vi "ProductionBoardReduction.vi"(11 "ProductionBoard":T3={"StartHour"=[{"Hour"=5, "Minute"=0}, {"Hour"=6, "Minute"=0}, {"Hour"=7, "Minute"=0}, {"Hour"=7, "Minute"=30}, {"Hour"=0, "Minute"=0}, {"Hour"=0, "Minute"=0}, {"Hour"=0, "Minute"=0}, {"Hour"=0, "Minute"=0}, {"Hour"=0, "Minute"=0}], "Goal"=[], "EndHour"=[{"Hour"=5, "Minute"=59}, {"Hour"=6, "Minute"=59}, {"Hour"=7, "Minute"=10}, {"Hour"=7, "Minute"=59}, {"Hour"=0, "Minute"=0}, {"Hour"=0, "Minute"=0}, {"Hour"=0, "Minute"=0}, {"Hour"=0, "Minute"=0}, {"Hour"=0, "Minute"=0}], "AM/PM"=[{"AM/PM"=0}, {"AM/PM"=0}, {"AM/PM"=0}, {"AM/PM"=0}, {"AM/PM"=0}, {"AM/PM"=0}, {"AM/PM"=0}, {"AM/PM"=0}, {"AM/PM"=0}], "Actual"=[], "%"=[], "Status"=[], "Comments"=[]} {"AM/PM"."AM/PM" items=["AM", "PM"]; "EndHour"."Minute" items=["00", "1", "2", "3", "4", "5", "6", "7", "8", "9", "10", "11", "12", "13", "14", "15", "16", "17", "18", "19", "20", "21", "22", "23", "24", "25", "26", "27", "28", "29", "30", "31", "32", "33", "34", "35", "36", "37", "38", "39", "40", "41", "42", "43", "44", "45", "46", "47", "48", "49", "50", "51", "52", "53", "54", "55", "56", "57", "58", "59"]; "EndHour"."Hour" items=["00", "1", "2", "3", "4", "5", "6", "7", "8", "9", "10", "11", "12", "13", "14", "15", "16", "17", "18", "19", "20", "21", "22", "23"]; "StartHour"."Minute" items=["00", "1", "2", "3", "4", "5", "6", "7", "8", "9", "10", "11", "12", "13", "14", "15", "16", "17", "18", "19", "20", "21", "22", "23", "24", "25", "26", "27", "28", "29", "30", "31", "32", "33", "34", "35", "36", "37", "38", "39", "40", "41", "42", "43", "44", "45", "46", "47", "48", "49", "50", "51", "52", "53", "54", "55", "56", "57", "58", "59"]; "StartHour"."Hour" items=["00", "1", "2", "3", "4", "5", "6", "7", "8", "9", "10", "11", "12", "13", "14", "15", "16", "17", "18", "19", "20", "21", "22", "23"]}) -> (3 "CloudProductionBoard":T2(array[cluster]) {"EndMinute" items=["00", "1", "2", "3", "4", "5", "6", "7", "8", "9", "10", "11", "12", "13", "14", "15", "16", "17", "18", "19", "20", "21", "22", "23", "24", "25", "26", "27", "28", "29", "30", "31", "32", "33", "34", "35", "36", "37", "38", "39", "40", "41", "42", "43", "44", "45", "46", "47", "48", "49", "50", "51", "52", "53", "54", "55", "56", "57", "58", "59"]; "EndHour" items=["00", "1", "2", "3", "4", "5", "6", "7", "8", "9", "10", "11", "12", "13", "14", "15", "16", "17", "18", "19", "20", "21", "22", "23"]; "InitialMinute" items=["00", "1", "2", "3", "4", "5", "6", "7", "8", "9", "10", "11", "12", "13", "14", "15", "16", "17", "18", "19", "20", "21", "22", "23", "24", "25", "26", "27", "28", "29", "30", "31", "32", "33", "34", "35", "36", "37", "38", "39", "40", "41", "42", "43", "44", "45", "46", "47", "48", "49", "50", "51", "52", "53", "54", "55", "56", "57", "58", "59"]; "InitialHour" items=["00", "1", "2", "3", "4", "5", "6", "7", "8", "9", "10", "11", "12", "13", "14", "15", "16", "17", "18", "19", "20", "21", "22", "23"]})   [LabVIEW 2017]
panel:
  out "ProductionHour":T1 {"EndMinute" items=["00", "1", "2", "3", "4", "5", "6", "7", "8", "9", "10", "11", "12", "13", "14", "15", "16", "17", "18", "19", "20", "21", "22", "23", "24", "25", "26", "27", "28", "29", "30", "31", "32", "33", "34", "35", "36", "37", "38", "39", "40", "41", "42", "43", "44", "45", "46", "47", "48", "49", "50", "51", "52", "53", "54", "55", "56", "57", "58", "59"]; "EndHour" items=["00", "1", "2", "3", "4", "5", "6", "7", "8", "9", "10", "11", "12", "13", "14", "15", "16", "17", "18", "19", "20", "21", "22", "23"]; "InitialMinute" items=["00", "1", "2", "3", "4", "5", "6", "7", "8", "9", "10", "11", "12", "13", "14", "15", "16", "17", "18", "19", "20", "21", "22", "23", "24", "25", "26", "27", "28", "29", "30", "31", "32", "33", "34", "35", "36", "37", "38", "39", "40", "41", "42", "43", "44", "45", "46", "47", "48", "49", "50", "51", "52", "53", "54", "55", "56", "57", "58", "59"]; "InitialHour" items=["00", "1", "2", "3", "4", "5", "6", "7", "8", "9", "10", "11", "12", "13", "14", "15", "16", "17", "18", "19", "20", "21", "22", "23"]}
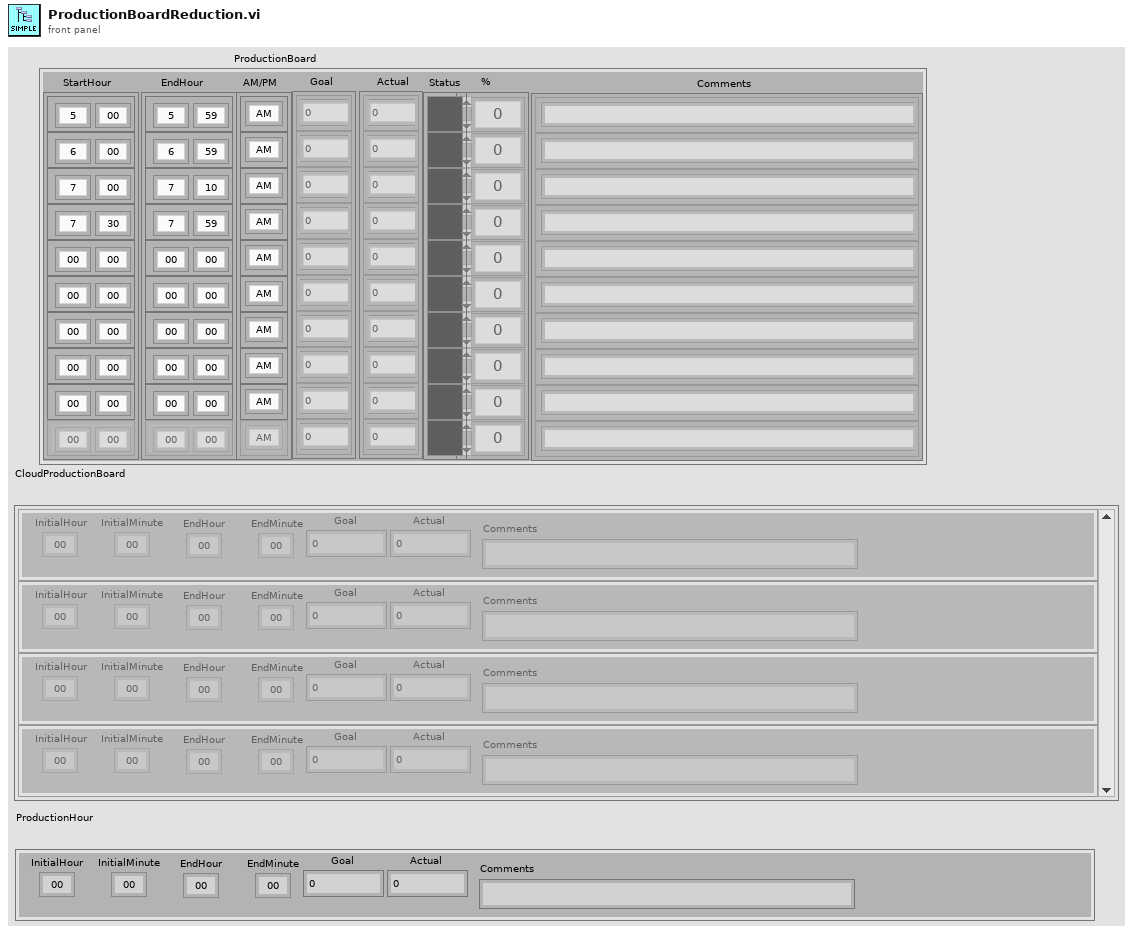
[diagram p1: front panel]
types:
  T1 = cluster{"InitialHour":u16, "InitialMinute":u16, "EndHour":u16, "EndMinute":u16, "Goal":dbl, "Actual":dbl, "Comments":string}
  T2 = cluster{"InitialHour":u16, "InitialMinute":u16, "EndHour":u16, "EndMinute":u16, "Goal":dbl, "Actual":dbl, "Comments":string}[]
  T3 = cluster{"StartHour":cluster{"Hour":u16, "Minute":u16}[], "Goal":cluster{"Goal":dbl}[], "EndHour":cluster{"Hour":u16, "Minute":u16}[], "AM/PM":cluster{"AM/PM":u16}[], "Actual":cluster{"Actual":dbl}[], "%":i32[], "Status":u32[], "Comments":cluster{"Comments":string}[]}
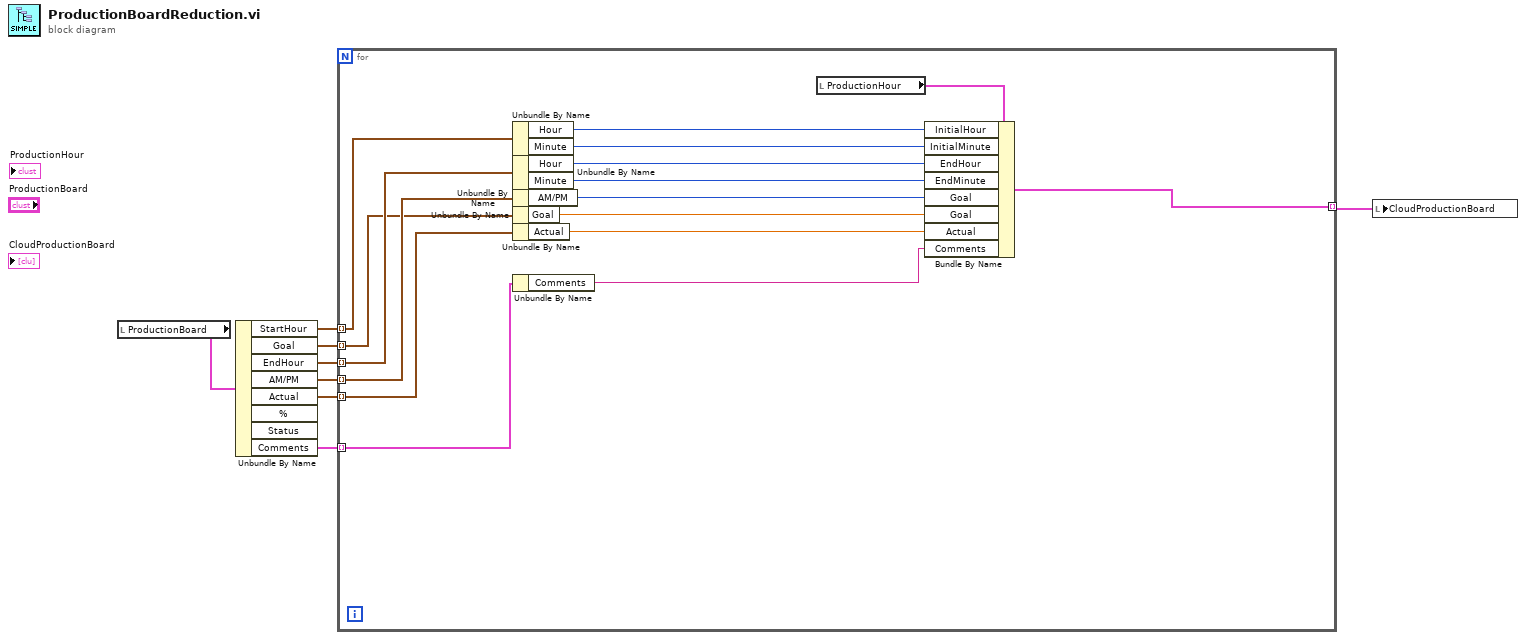
[diagram p0: block diagram]
diagram:
  n1 = local read "ProductionBoard"() -> (w8:T3)
  n2 = Unbundle By Name(w8) -> ("StartHour"=w7:cluster{"Hour":u16, "Minute":u16}[], "Goal"=w6:cluster{"Goal":dbl}[], "EndHour"=w5:cluster{"Hour":u16, "Minute":u16}[], "AM/PM"=w4:cluster{"AM/PM":u16}[], "Actual"=w3:cluster{"Actual":dbl}[], "Comments"=w2:cluster{"Comments":string}[])  [unwired: 2 out]
  n3 = for {
    tunnel: w7 -> [w24] mode=indexing
    tunnel: w6 -> [w15] mode=indexing
    tunnel: w5 -> [w20] mode=indexing
    tunnel: w4 -> [w18] mode=indexing
    tunnel: w3 -> [w14] mode=indexing
    tunnel: w2 -> [w11] mode=indexing
    tunnel: [w10] -> w1 mode=indexing
    n4 = Unbundle By Name(w24) -> ("Hour"=w22:u16, "Minute"=w21:u16)
    n5 = Unbundle By Name(w20) -> ("Hour"=w19:u16, "Minute"=w16:u16)
    n6 = Unbundle By Name(w18) -> ("AM/PM"=w17:u16)
    n7 = Unbundle By Name(w15) -> ("Goal"=w12:dbl)
    n8 = Unbundle By Name(w14) -> ("Actual"=w13:dbl)
    n9 = Unbundle By Name(w11) -> ("Comments"=w9:string)
    n10 = local read "ProductionHour"() -> (w23:T1)
    n11 = Bundle By Name(cluster=w23, "InitialHour"=w22, "InitialMinute"=w21, "EndHour"=w19, "EndMinute"=w16, "Goal"=w17, "Goal"=w12, "Actual"=w13, "Comments"=w9) -> (w10:T1)
  }
  n12 = local write "CloudProductionBoard"(w1) -> ()
